vi "Data Analysis.vi"(0 "Data In":string="AD 2E 92 00 D8 03 92 01 AD 2E 00 00 D8 03 26 02 AD 2E 00 00 D8 03 92 01 00 00 00 00 D0 07 AA 55 AA 55 06 1E 24 AA AD 2E 92 00 D8 03 92 01 AD 2E 00 00 D8 03 26 02 AD 2E 00 00 D8 03 92 01 00 00 00 00 D0 07 AA 55 AA 55 06 1E 88 AA AD 2E 92 00 13 00 92 01 A8 30 09 00 13 00 92 01 AD 2E 09 00 13 00 92 01 00 00 00 00 56 06 AA 55 AA 55 06 1E 88 AA AD 2E 92 00 13 00 92 01 A8 30 09 00 13 00 92 01 AD 2E 09 00 13 00 92 01 00 00 00 00 56 06 AA 55 ", 11 "error in":errorcluster) -> (1 "APOS_Voltage":dbl, 2 "DPOS_Voltage":dbl, 3 "ANEG_Voltage":dbl, 12 "APOS_Temperature":dbl, 13 "ANEG_Temperature":dbl, 14 "DPOS_Temperature":dbl, 15 "error out":errorcluster)   [LabVIEW 2020]
uses:
  <vilib>/regexp/Match Regular Expression.xnode
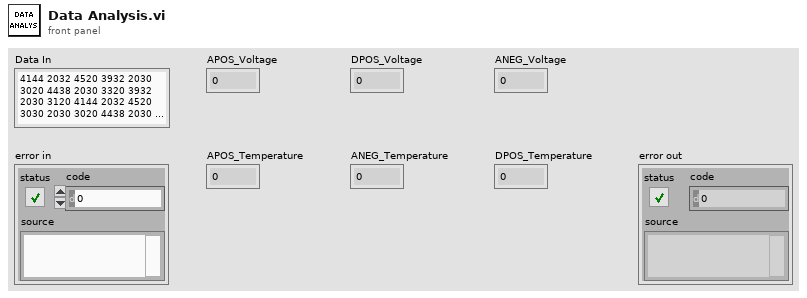
[diagram p1: front panel]
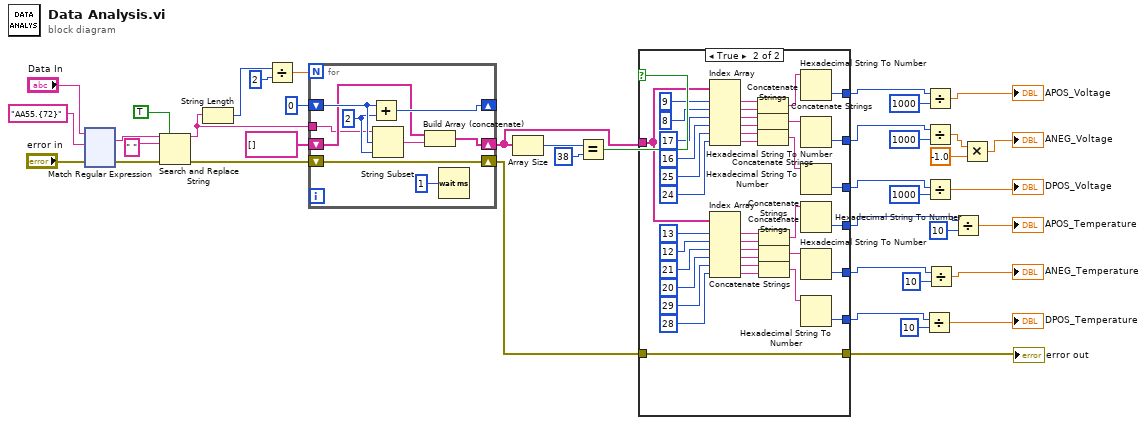
[diagram p0: block diagram]
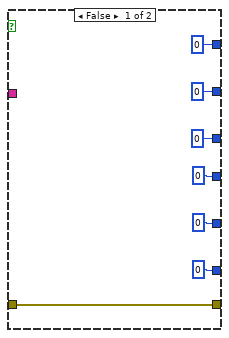
[diagram p2: hidden frame]
diagram:
  n1 = xnode "Match Regular Expression"("input string"="Data In", "regular expression"="AA55.{72}", "error in"="error in") -> ("whole match"=w30:string, "error out"=w24:errorcluster)  [unwired: 3 in, 3 out]
  n2 = Search and Replace String(replace all?=TRUE ("replace all? (F)"), input string=w30, search string=" ", error in=w24) -> (result string=w34:string, error out=w23:errorcluster)  [unwired: 4 in, 2 out]
  n3 = String Length(string=w34) -> (length=w33:i32)
  n4 = Divide(x=w33, y=2) -> (x/y=w31:dbl)
  n5 = for {
    N: w31 -> [_]
    shift-right: [w48] -> _
    shift-left: 0 -> [w49]
    shift-right: [w44] -> w26
    shift-left: string[] [] -> [w45]
    tunnel: w34 -> [w42]
    shift-right: [w41] -> w22
    shift-left: w23 -> [w41]
    w47 = 2 ("length (rest)")
    n6 = Add(x=w49, y=w47) -> (x+y=w48:i32)
    n7 = String Subset(string=w42, offset (0)=w49, length (rest)=w47) -> (substring=w46:string)
    n8 = Build Array (concatenate)(w45, w46) -> (w44:string[])
    n9 = Wait (ms)(milliseconds to wait=u32 1) -> ()  [unwired: 1 out]
  }
  n10 = Array Size(array=w26) -> (size(s)=w29:i32)
  n11 = Equal?(x=w29, y=38) -> (x = y?=w27:bool)
  n12 = case shown="True" w27 {
    tunnel: w26 -> [_ w70]
    tunnel: [u32 0 w63] -> w18
    tunnel: [u32 0 w62] -> w19
    tunnel: [u32 0 w61] -> w20
    tunnel: [u32 0 w60] -> w9
    tunnel: [u32 0 w59] -> w10
    tunnel: [u32 0 w58] -> w11
    tunnel: w22 -> [w50 w57]
    tunnel: [w50 w57] -> w21
    frame False {
    }
    frame True {
      n13 = Index Array(array=w70, index #1=9 ("index"), index #2=8 ("index"), index #3=17 ("index"), index #4=16 ("index"), index #5=25 ("index"), index #6=24 ("index")) -> (element #1=w88:string, element #2=w87:string, element #3=w86:string, element #4=w85:string, element #5=w84:string, element #6=w83:string)
      n14 = Index Array(array=w70, index #1=13 ("index"), index #2=12 ("index"), index #3=21 ("index"), index #4=20 ("index"), index #5=29 ("index"), index #6=28 ("index")) -> (element #1=w77:string, element #2=w78:string, element #3=w79:string, element #4=w80:string, element #5=w81:string, element #6=w82:string)
      n15 = Concatenate Strings(w88, w87) -> (w69:string)
      n16 = Concatenate Strings(w86, w85) -> (w68:string)
      n17 = Concatenate Strings(w84, w83) -> (w67:string)
      n18 = Concatenate Strings(w77, w78) -> (w66:string)
      n19 = Concatenate Strings(w79, w80) -> (w65:string)
      n20 = Concatenate Strings(w81, w82) -> (w64:string)
      n21 = Hexadecimal String To Number(string=w69) -> (number=w58:u32)  [unwired: 2 in, 1 out]
      n22 = Hexadecimal String To Number(string=w68) -> (number=w59:u32)  [unwired: 2 in, 1 out]
      n23 = Hexadecimal String To Number(string=w67) -> (number=w60:u32)  [unwired: 2 in, 1 out]
      n24 = Hexadecimal String To Number(string=w66) -> (number=w61:u32)  [unwired: 2 in, 1 out]
      n25 = Hexadecimal String To Number(string=w65) -> (number=w62:u32)  [unwired: 2 in, 1 out]
      n26 = Hexadecimal String To Number(string=w64) -> (number=w63:u32)  [unwired: 2 in, 1 out]
    }
  }
  "error out" <- w21
  n27 = Divide(x=w18, y=u32 10) -> (x/y=→"DPOS_Temperature":dbl)
  n28 = Divide(x=w11, y=u32 1000) -> (x/y=→"APOS_Voltage":dbl)
  n29 = Divide(x=w10, y=u32 1000) -> (x/y=w3:dbl)
  n30 = Divide(x=w9, y=u32 1000) -> (x/y=→"DPOS_Voltage":dbl)
  n31 = Divide(x=w19, y=u32 10) -> (x/y=→"ANEG_Temperature":dbl)
  n32 = Divide(x=w20, y=u32 10) -> (x/y=→"APOS_Temperature":dbl)
  n33 = Multiply(x=w3, y=-1.0) -> (x*y=→"ANEG_Voltage":dbl)
